vi "GetInnerXMLTag.vi"(1 "String":string) -> (0 "Value":string)   [LabVIEW 2012]
doc: "Looks for all closing XML tags and finds their opening tags. Returns the value of the innermost XML tag."
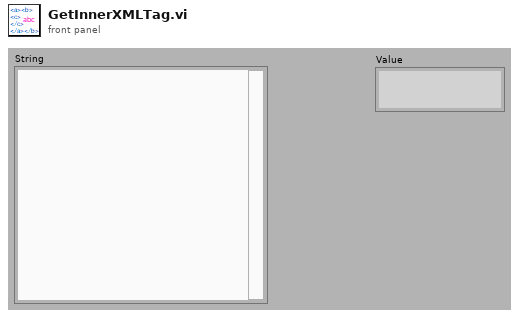
[diagram p1: front panel]
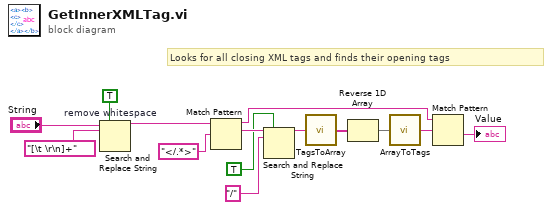
[diagram p0: block diagram]
diagram:
  # "Looks for all closing XML tags and finds their opening tags"
  n1 = Search and Replace String "remove whitespace"(replace all?=TRUE ("replace all? (F)"), input string="String", search string="[\t \r\n]+") -> (result string=w3:string)  [unwired: 5 in, 3 out]
  n2 = Match Pattern(string=w3, regular expression="</.*>") -> (before substring=w10:string, match substring=w13:string)  [unwired: 1 in, 2 out]
  n3 = Search and Replace String(replace all?=TRUE ("replace all? (F)"), input string=w13, search string="/") -> (result string=w8:string)  [unwired: 5 in, 3 out]
  n4 = call <userlib>:"TagsToArray.vi"("Tags"=w8) -> ("Array"=w7:string[])
  n5 = Reverse 1D Array(array=w7) -> (reversed array=w6:string[])
  n6 = call <userlib>:"ArrayToTags.vi"("Array"=w6) -> ("String"=w5:string)
  n7 = Match Pattern(string=w10, regular expression=w5) -> (after substring=→"Value":string)  [unwired: 1 in, 3 out]
